vi "piezoUSBRead.vi"() -> (0 "piezoPosition":dbl)   [LabVIEW 2017]
uses:
  globalDevices.vi
  Piezo/lvlib/Madlib.lvlib
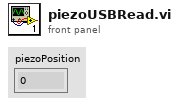
[diagram p1: front panel]
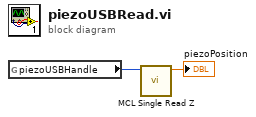
[diagram p0: block diagram]
diagram:
  n1 = global read "globalDevices.vi" "piezoUSBHandle"() -> (w2:i32)
  n2 = call "MCL Single Read Z.vi"("handle"=w2) -> ("function return"=→"piezoPosition":dbl)  [unwired: 10 in]
